vi "PAN_GetCommModsInfo.vi"(8 "errors":errorcluster[](array[cluster]), 10 "coms to run":path[](array[path]), 11 "configfile":path) -> (0 "error out":errorcluster, 2 "info":string)   [LabVIEW 2016]
uses:
  <vilib>/Utility/config.llb/Read Key (String).vi
  <vilib>/Utility/config.llb/NI_LVConfig.lvlib
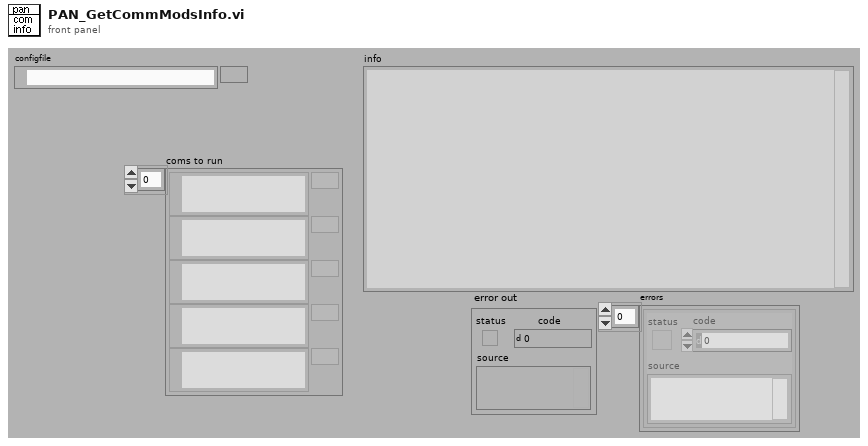
[diagram p1: front panel]
types:
  T1 = typedef "NI_LVConfig.lvlib/Config Data RefNum.ctl" = refnum<k1>
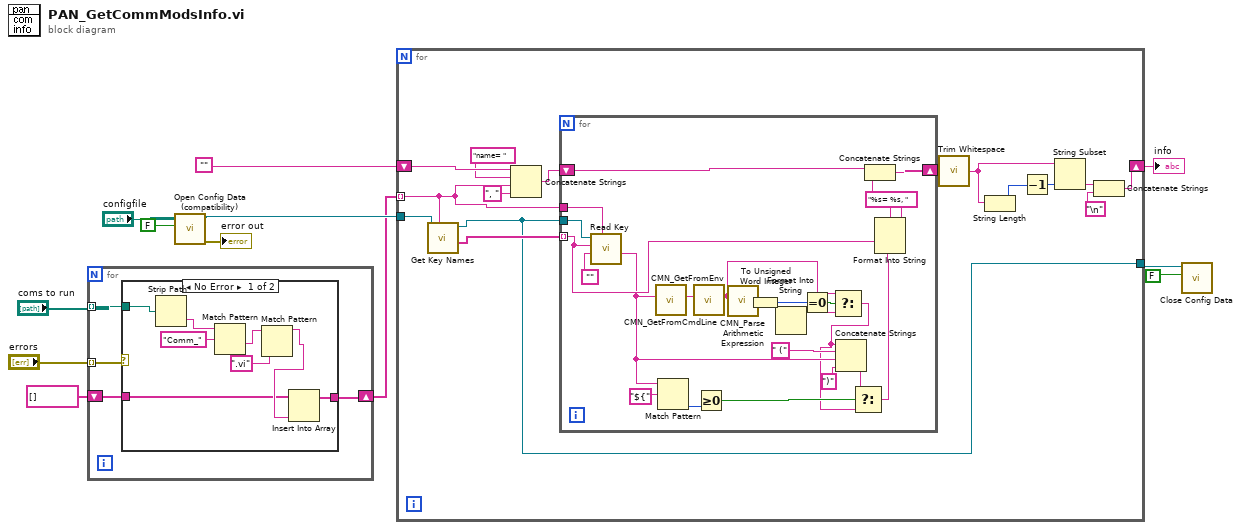
[diagram p0: block diagram]
diagram:
  n1 = for {
    tunnel: "coms to run" -> [w16] mode=indexing
    tunnel: "errors" -> [w15] mode=indexing
    shift-right: [w14] -> w2
    shift-left: string[] [] -> [w13]
    n2 = case shown="No Error" w15 {
      tunnel: w16 -> [w24 _]
      tunnel: [w18 w25] -> w14
      tunnel: w13 -> [w17 w25]
      frame No Error {
        n3 = Strip Path(path=w24) -> (name=w23:string)  [unwired: 1 out]
        n4 = Match Pattern(string=w23, regular expression="Comm_") -> (after substring=w21:string)  [unwired: 4 out]
        n5 = Match Pattern(string=w21, regular expression=".vi") -> (before substring=w19:string)  [unwired: 4 out]
        n6 = Insert Into Array(array=w17, new element=w19) -> (w18:string[])  [unwired: 1 in]
      }
      frame Error {
      }
    }
  }
  n7 = call <vilib>:"Open Config Data (compatibility).vi"("create file if necessary (T)"=FALSE ("create file if necessary? (T)"), "configuration file path"="configfile") -> ("error out"=→"error out":errorcluster, "refnum"=w7:T1)  [unwired: 7 in, 1 out]
  n8 = for {
    tunnel: w7 -> [w38]
    shift-right: [w39] -> w9
    shift-left: "" -> [w40]
    tunnel: w2 -> [w30] mode=indexing
    tunnel: [w26] -> w5
    n9 = call <vilib>:"Get Key Names.vi"("section"=w30, "refnum"=w38) -> ("key names"=w37:string[], "refnum out"=w26:T1)  [unwired: 1 in, 7 out]
    n10 = Concatenate Strings(w40, "name= " ("string"), w30, ", " ("string")) -> (w34:string)
    n11 = for {
      tunnel: w37 -> [w60] mode=indexing
      shift-right: [w56] -> w29
      shift-left: w34 -> [w57]
      tunnel: w30 -> [w63]
      tunnel: w26 -> [w62]
      n12 = call-poly <vilib>:"Read Key.vi"("section"=w63, "default value"="", "key"=w60, "refnum"=w62) -> ("value"=w49:string)  [unwired: 2 in, 5 out]
      n13 = call "CMN_GetFromCmdLine.vi"("str in"=w49) -> ("str out"=w55:string)  [unwired: 10 out]
      n14 = Match Pattern(string=w49, regular expression="${" ("x")) -> (offset past match=w54:i32)  [unwired: 4 out]
      n15 = call "CMN_GetFromEnv.vi"("str in"=w55) -> ("str out"=w45:string)  [unwired: 10 out]
      n16 = Greater Or Equal To 0?(x=w54) -> (x >= 0?=w52:bool)
      n17 = call "CMN_Parse Arithmetic Expression.vi"("Arithmetic Expression"=w45) -> ("Result"=w44:dbl)
      n18 = To Unsigned Word Integer(number=w44) -> (unsigned 16bit integer=w41:u16)
      n19 = Format Into String(w41) -> (resulting string=w43:string)  [unwired: 3 in, 1 out]
      n20 = Equal To 0?(x=w41) -> (x = 0?=w46:bool)
      n21 = Select(t=w45, s=w46, f=w43) -> (s? t:f=w42:string)
      n22 = Concatenate Strings(w42, " (" ("string"), w49, ")" ("string")) -> (w48:string)
      n23 = Select(t=w48, s=w52, f=w42) -> (s? t:f=w47:string)
      n24 = Format Into String(format string="%s= %s, ", w60, w47) -> (resulting string=w58:string)  [unwired: 2 in, 1 out]
      n25 = Concatenate Strings(w57, w58) -> (w56:string)
    }
    n26 = call <vilib>:"Trim Whitespace.vi"("string"=w29) -> ("trimmed string"=w27:string)  [unwired: 1 in]
    n27 = String Length(string=w27) -> (length=w33:i32)
    n28 = Decrement(x=w33) -> (x-1=w32:i32)
    n29 = String Subset(string=w27, length (rest)=w32) -> (substring=w28:string)  [unwired: 1 out]
    n30 = Concatenate Strings(w28, "\n") -> (w39:string)
  }
  "info" <- w9
  n31 = call <vilib>:"Close Config Data.vi"("write file if changed (T)"=FALSE ("write configuration file? (T)"), "refnum"=w5) -> ()  [unwired: 1 in, 9 out]
